vi "글로벌 2.vi"() -> ()   [LabVIEW 2014]
panel:
  in  "정지":bool
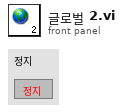
[diagram p1: front panel]
diagram:
